vi "ReadExpectedDependencies.vi"(8 "error in (no error)":errorcluster, 11 "Library Name":string) -> (0 "error out":errorcluster, 1 "ExpectedDeps Path":path, 2 "Found?":bool, 3 "ExpectedDependencies":string[](array[string]))   [LabVIEW 2023, in "DepsWatch.lvlib"]
uses:
  DepsWatch.lvlib
  <vilib>/Utility/config.llb/NI_LVConfig.lvlib
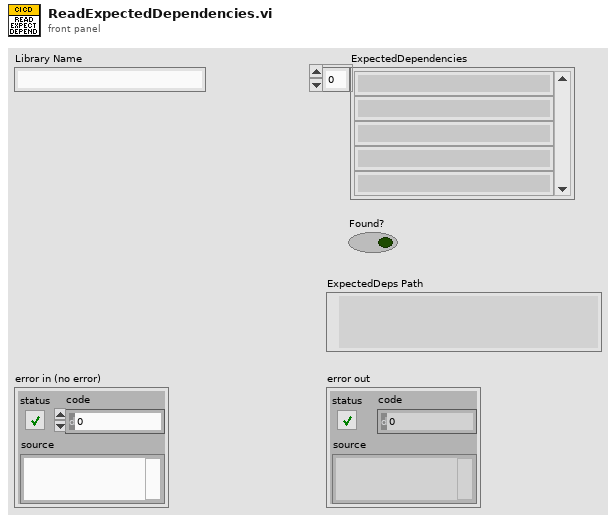
[diagram p1: front panel]
types:
  T1 = typedef "NI_LVConfig.lvlib/Config Data RefNum.ctl" = refnum<k1>
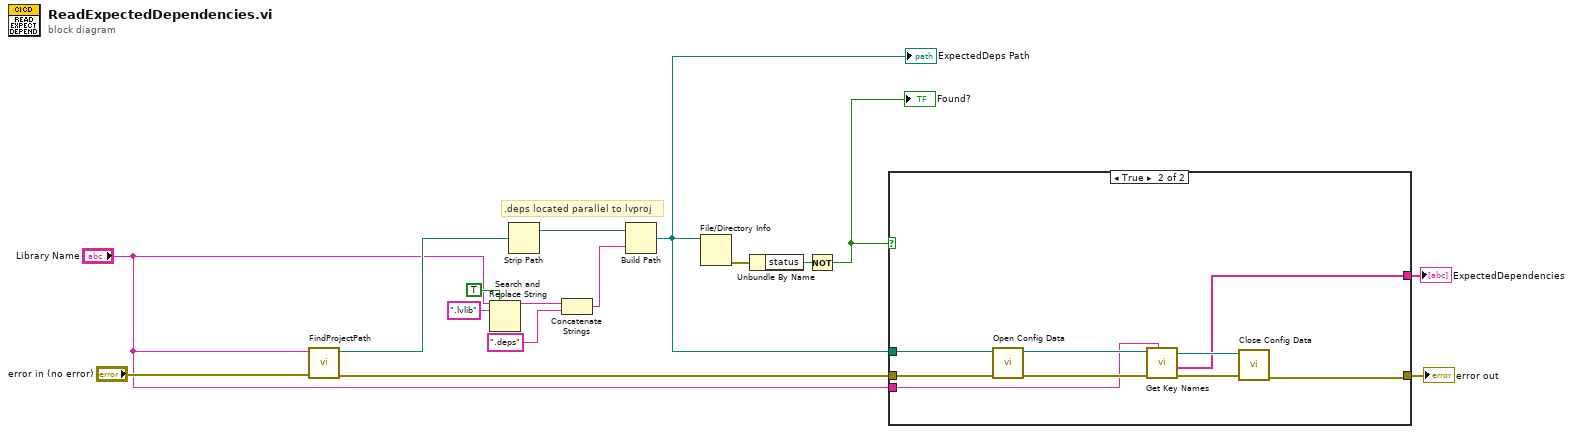
[diagram p0: block diagram]
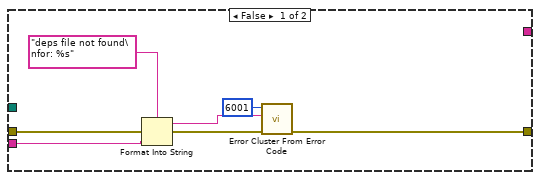
[diagram p2: hidden frame]
diagram:
  # ".deps located parallel to lvproj"
  n1 = call "FindProjectPath.vi"("error in (no error)"="error in (no error)", "Library Name"="Library Name") -> ("error out"=w8:errorcluster, "Project Path"=w15:path)  [unwired: 7 in, 1 out]
  n2 = Search and Replace String(replace all?=TRUE ("replace all? (F)"), input string="Library Name", search string=".lvlib") -> (result string=w11:string)  [unwired: 5 in, 3 out]
  n3 = Strip Path(path=w15) -> (stripped path=w14:path)  [unwired: 1 out]
  n4 = Concatenate Strings(w11, ".deps" ("string")) -> (w9:string)
  n5 = Build Path(base path=w14, name or relative path=w9) -> (appended path=w5:path)
  "ExpectedDeps Path" <- w5
  n6 = File/Directory Info(path=w5) -> (error out=w1:errorcluster)  [unwired: 1 in, 6 out]
  n7 = Unbundle By Name(w1) -> ("status"=w2:bool)
  n8 = Not(x=w2) -> (.not. x?=w4:bool)
  "Found?" <- w4
  n9 = case shown="True" w4 {
    tunnel: w8 -> [w22 w32]
    tunnel: "Library Name" -> [w20 w28]
    tunnel: [w17 w24] -> w7
    tunnel: w5 -> [_ w31]
    tunnel: [_ w25] -> w6
    frame False {
      n10 = Format Into String(format string="deps file not found\nfor: %s" ("error message (\"\")"), error in=w22, w20) -> (resulting string=w19:string, error out=w18:errorcluster)  [unwired: 1 in]
      n11 = call <vilib>:"Error Cluster From Error Code.vi"("error in (no error)"=w18, "error message (\"\")"=w19, "error code (0)"=6001) -> ("error out"=w17:errorcluster)  [unwired: 6 in]
    }
    frame True {
      n12 = call <vilib>:"Open Config Data.vi"("error in (no error)"=w32, "configuration file path"=w31) -> ("error out"=w30:errorcluster, "refnum"=w29:T1)  [unwired: 7 in, 1 out]
      n13 = call <vilib>:"Get Key Names.vi"("section"=w28, "error in (no error)"=w30, "refnum"=w29) -> ("error out"=w27:errorcluster, "key names"=w25:string[], "refnum out"=w26:T1)  [unwired: 5 in, 1 out]
      n14 = call <vilib>:"Close Config Data.vi"("error in (no error)"=w27, "refnum"=w26) -> ("error out"=w24:errorcluster)  [unwired: 8 in, 1 out]
    }
  }
  "error out" <- w7
  "ExpectedDependencies" <- w6
